vi "FastBeamMode.vi"() -> ()   [LabVIEW 2021]
uses:
  D:/tmytek/Source/bbox-api/example/BBoxOne Series/LabVIEW/BBoxAPI.dll
  BBoxAPI.dll
  Kernel32.dll
panel:
  out "Console Log":string
  out "ScanningDevice":string[](array[string])
  out "Target AAKit Name":string
  out "selectAAKit":i32(ring)=13 items=["OK"=0, "WARNING"=1, "ERROR"=2, "NO_RESPONSE"=3, "ERROR_GET_SN"=10, "ERROR_DEV_TYPE"=11, "ERROR_INIT_OBJECT"=12, "ERROR_DEV_NOT_INIT"=13, "ERROR_METHOD_NOT_FOUND"=14, "ERROR_REFLECTION"=15, "ERROR_POWER"=16, "ERROR_NETWORK_NOT_INIT"=20, "ERROR_NETWORK_INIT"=21, "ERROR_NETWORK_CONNECT_TIMEOUT"=22, "ERROR_DISCONNECT"=23, "ERROR_SOCKET"=24, "ERROR_SEND_CMD"=25, "ERROR_RESP_CMD"=26, "ERROR_DEV_COUNT_ZERO"=30, "ERROR_CMD"=40, "ERROR_CMD_INIT"=41, "ERROR_BF_AAKIT"=100, "ERROR_BF_NO_AAKIT"=101, "ERROR_BF_CALI_PATH"=102, "ERROR_BF_BEAMXY"=103, "ERROR_BF_GEN"=104, "ERROR_BF_TRMODE"=105, "STATUS_BF_LOAD_CALI_INCOMPLTE"=106, "ERROR_BF_LOAD_CALI_PARSE_FAILED"=107, "ERROR_FREQ_EQUATION"=250, "ERROR_PLO_CRC"=251, "WARNING_HARMONIC"=252, "ERROR_HARMONIC_BLOCK"=253]
  out "checkCaliTableLocation":bool
  in  "Fast BeamMode Enable":bool=TRUE
  out "getAAKitList":string[](array[string])
  out "getFrequencyList":string[](array[string])
  in  "Target AAKit Index":i32 min=1 max=2 step=1
  in  "Target Freq Index":i32 min=1 max=2 step=1
  out "setOperatingFreq":i32(ring)=13 items=["OK"=0, "WARNING"=1, "ERROR"=2, "NO_RESPONSE"=3, "ERROR_GET_SN"=10, "ERROR_DEV_TYPE"=11, "ERROR_INIT_OBJECT"=12, "ERROR_DEV_NOT_INIT"=13, "ERROR_METHOD_NOT_FOUND"=14, "ERROR_REFLECTION"=15, "ERROR_POWER"=16, "ERROR_NETWORK_NOT_INIT"=20, "ERROR_NETWORK_INIT"=21, "ERROR_NETWORK_CONNECT_TIMEOUT"=22, "ERROR_DISCONNECT"=23, "ERROR_SOCKET"=24, "ERROR_SEND_CMD"=25, "ERROR_RESP_CMD"=26, "ERROR_DEV_COUNT_ZERO"=30, "ERROR_CMD"=40, "ERROR_CMD_INIT"=41, "ERROR_BF_AAKIT"=100, "ERROR_BF_NO_AAKIT"=101, "ERROR_BF_CALI_PATH"=102, "ERROR_BF_BEAMXY"=103, "ERROR_BF_GEN"=104, "ERROR_BF_TRMODE"=105, "STATUS_BF_LOAD_CALI_INCOMPLTE"=106, "ERROR_BF_LOAD_CALI_PARSE_FAILED"=107, "ERROR_FREQ_EQUATION"=250, "ERROR_PLO_CRC"=251, "WARNING_HARMONIC"=252, "ERROR_HARMONIC_BLOCK"=253]
  out "SN":string
  out "Set_Fast_Parallel_Mode":i32(ring) items=["OK"=0, "WARNING"=1, "ERROR"=2, "NO_RESPONSE"=3, "ERROR_GET_SN"=10, "ERROR_DEV_TYPE"=11, "ERROR_INIT_OBJECT"=12, "ERROR_DEV_NOT_INIT"=13, "ERROR_METHOD_NOT_FOUND"=14, "ERROR_REFLECTION"=15, "ERROR_POWER"=16, "ERROR_SCAN_NOT_FOUND"=17, "ERROR_UNMATCH_RETURN_TYPE"=18, "ERROR_NETWORK_NOT_INIT"=20, "ERROR_NETWORK_INIT"=21, "ERROR_NETWORK_CONNECT_TIMEOUT"=22, "ERROR_DISCONNECT"=23, "ERROR_SOCKET"=24, "ERROR_SEND_CMD"=25, "ERROR_RESP_CMD"=26, "ERROR_DEV_COUNT_ZERO"=30, "ERROR_DEV_DUMMY_FUNC"=31, "ERROR_CMD"=40, "ERROR_CMD_INIT"=41, "ERROR_BF_AAKIT"=100, "ERROR_BF_NO_AAKIT"=101, "ERROR_BF_CALI_PATH"=102, "ERROR_BF_BEAMXY"=103, "ERROR_BF_GEN"=104, "ERROR_BF_TRMODE"=105, "STATUS_BF_LOAD_CALI_INCOMPLTE"=106, "ERROR_BF_LOAD_CALI_PARSE_FAILED"=107, "ERROR_BF_UNLOAD_CALI"=108, "ERROR_BF_CALI_VERSION_UNSUPPORTED"=109, "ERROR_BF_CALI_DATA_NOT_FOUND"=110, "ERROR_FREQ_EQUATION"=250, "ERROR_PLO_CRC"=251, "WARNING_HARMONIC"=252, "ERROR_HARMONIC_BLOCK"=253, "ERROR_FW_UPGRADE_IP_INVALID"=300, "ERROR_FW_VERSION_NOT_SUPPORT"=301]
  out "Init":i32(ring)=13 items=["OK"=0, "WARNING"=1, "ERROR"=2, "NO_RESPONSE"=3, "ERROR_GET_SN"=10, "ERROR_DEV_TYPE"=11, "ERROR_INIT_OBJECT"=12, "ERROR_DEV_NOT_INIT"=13, "ERROR_METHOD_NOT_FOUND"=14, "ERROR_REFLECTION"=15, "ERROR_POWER"=16, "ERROR_NETWORK_NOT_INIT"=20, "ERROR_NETWORK_INIT"=21, "ERROR_NETWORK_CONNECT_TIMEOUT"=22, "ERROR_DISCONNECT"=23, "ERROR_SOCKET"=24, "ERROR_SEND_CMD"=25, "ERROR_RESP_CMD"=26, "ERROR_DEV_COUNT_ZERO"=30, "ERROR_CMD"=40, "ERROR_CMD_INIT"=41, "ERROR_BF_AAKIT"=100, "ERROR_BF_NO_AAKIT"=101, "ERROR_BF_CALI_PATH"=102, "ERROR_BF_BEAMXY"=103, "ERROR_BF_GEN"=104, "ERROR_BF_TRMODE"=105, "STATUS_BF_LOAD_CALI_INCOMPLTE"=106, "ERROR_BF_LOAD_CALI_PARSE_FAILED"=107, "ERROR_FREQ_EQUATION"=250, "ERROR_PLO_CRC"=251, "WARNING_HARMONIC"=252, "ERROR_HARMONIC_BLOCK"=253]
  in  "Start":bool=TRUE
  in  "Set Current Working Directory":path
  out "Get Current Working Directory":path
  out "Exists Table Filenames":string[](array[string])
  # "Notice:\n\nThe Set / Get Current Working Diectory Path must be the sample code directory path : bbox-api\\example\\BBoxOne Series\\LabVIEW\\\n\nMust exist\n\n1. bbox-api\\example\\BBoxOne Series\\LabVIEW\\BBoxAPI.dll\n\n2. bbox-api\\example\\BBoxOne Series\\LabVIEW\\files\\\n\n3. bbox-api\\example\\BBoxOne Series\\LabVIEW\\logs\\"
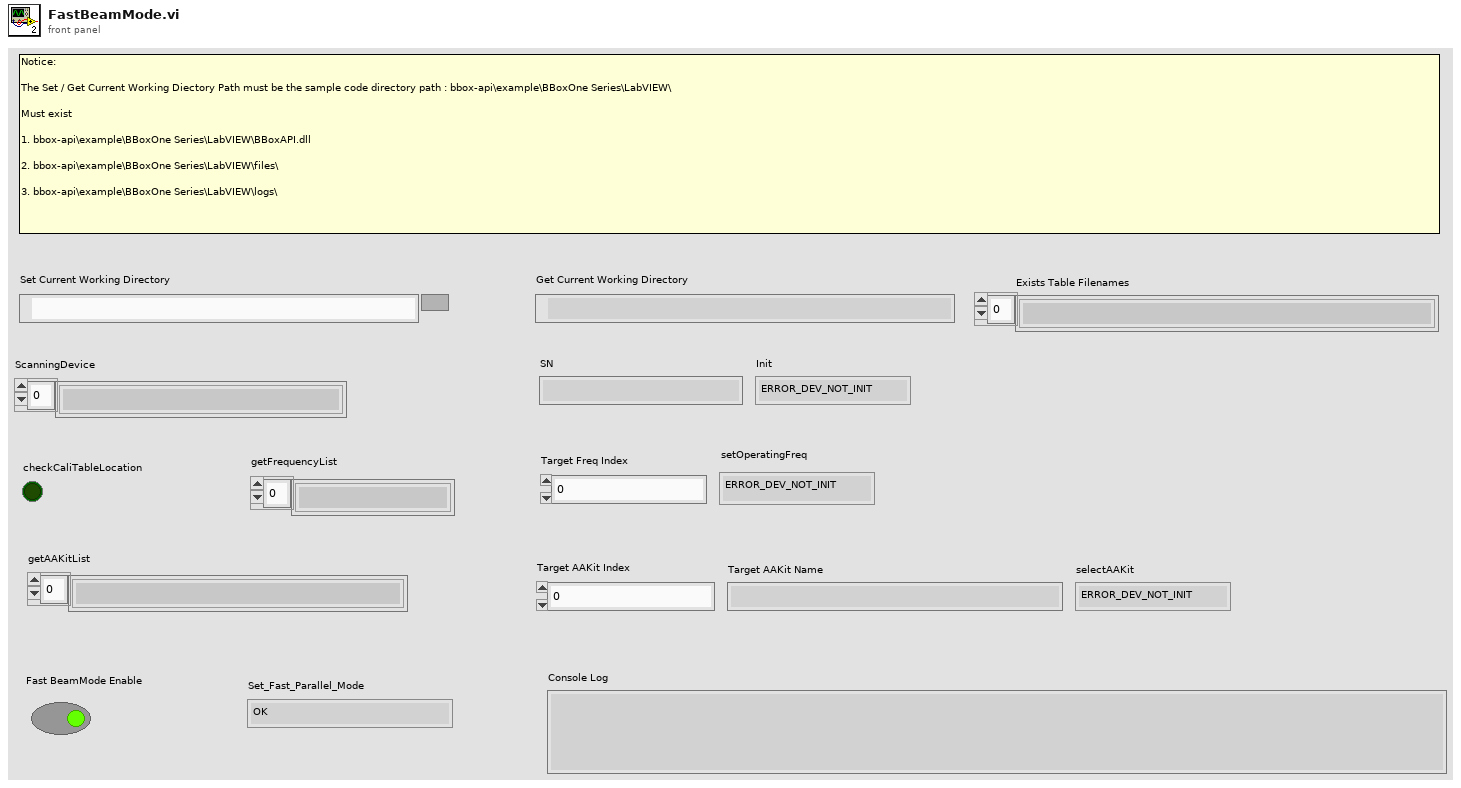
[diagram p1: front panel]
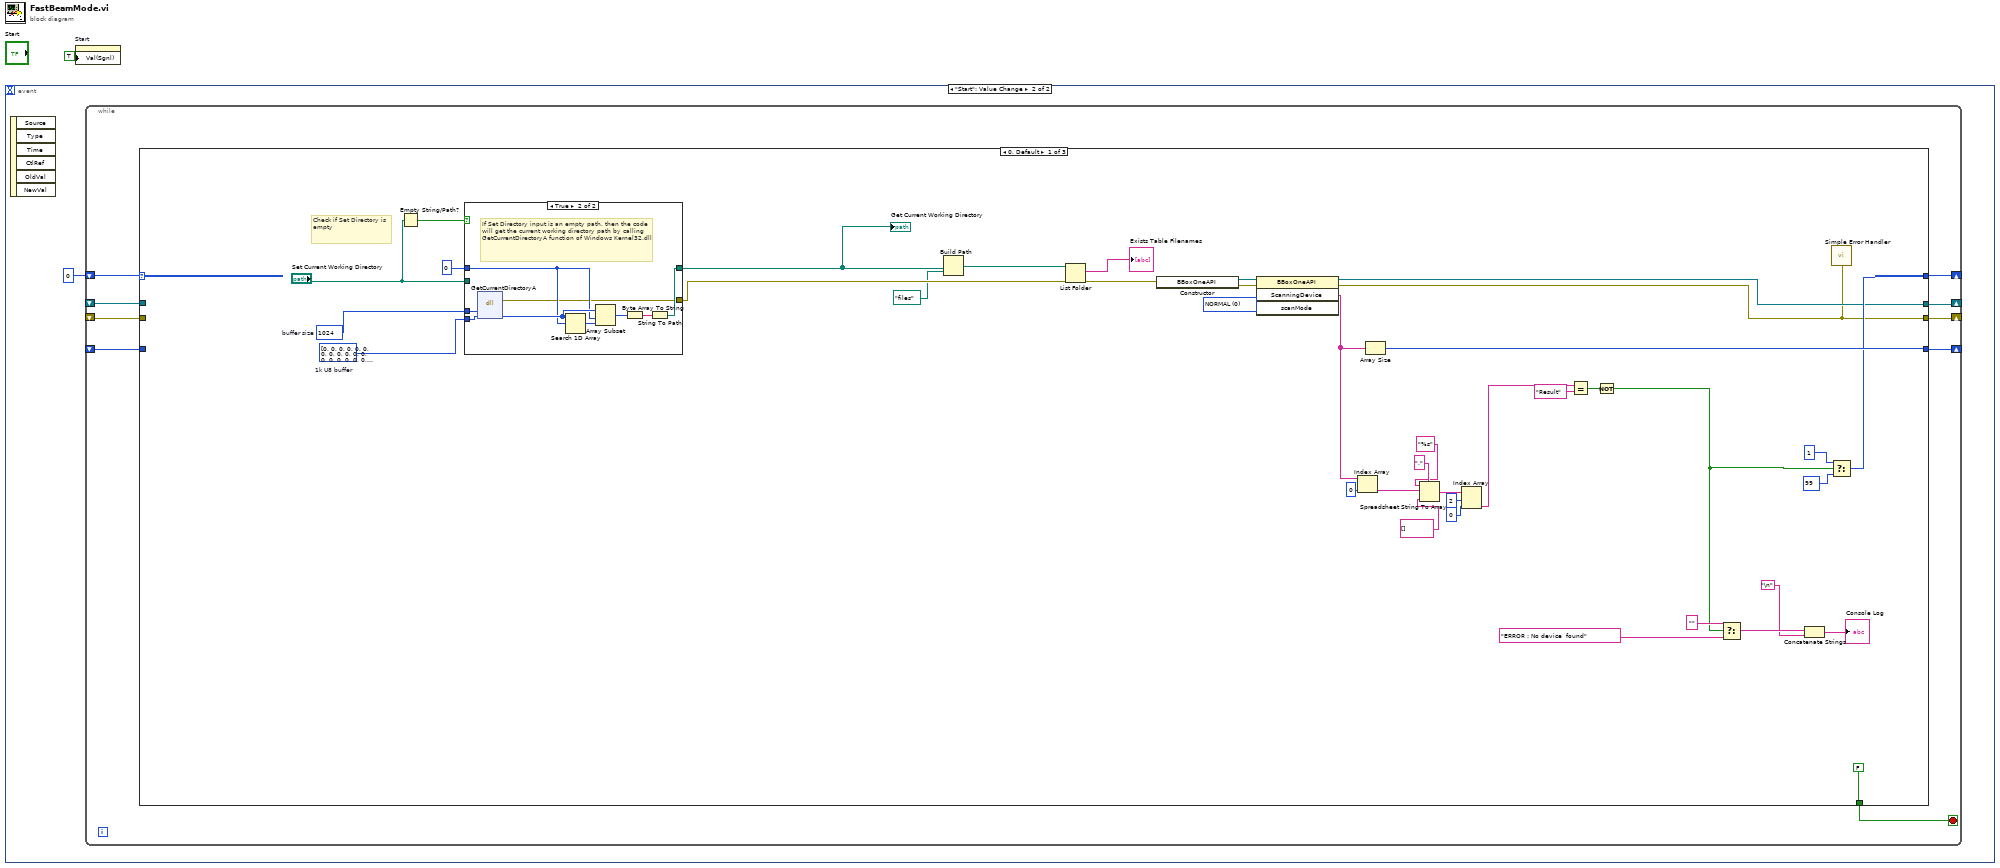
[diagram p0: block diagram]
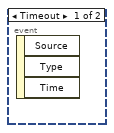
[diagram p2: hidden frame]
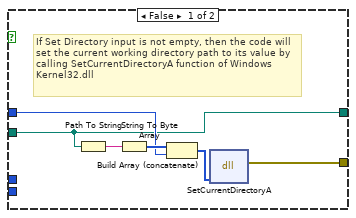
[diagram p3: hidden frame]
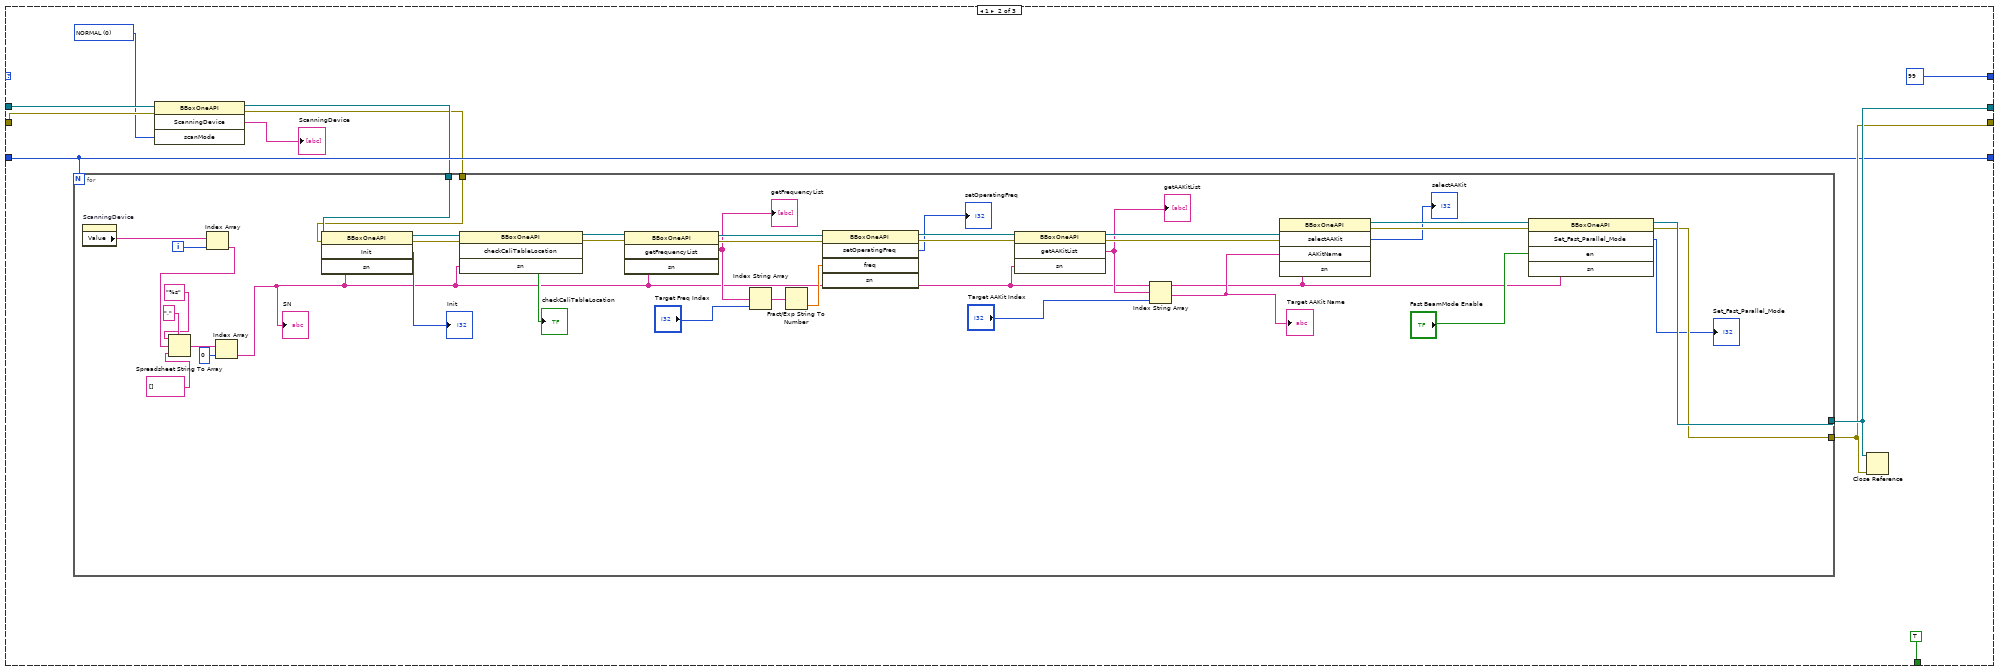
[diagram p4: hidden frame]
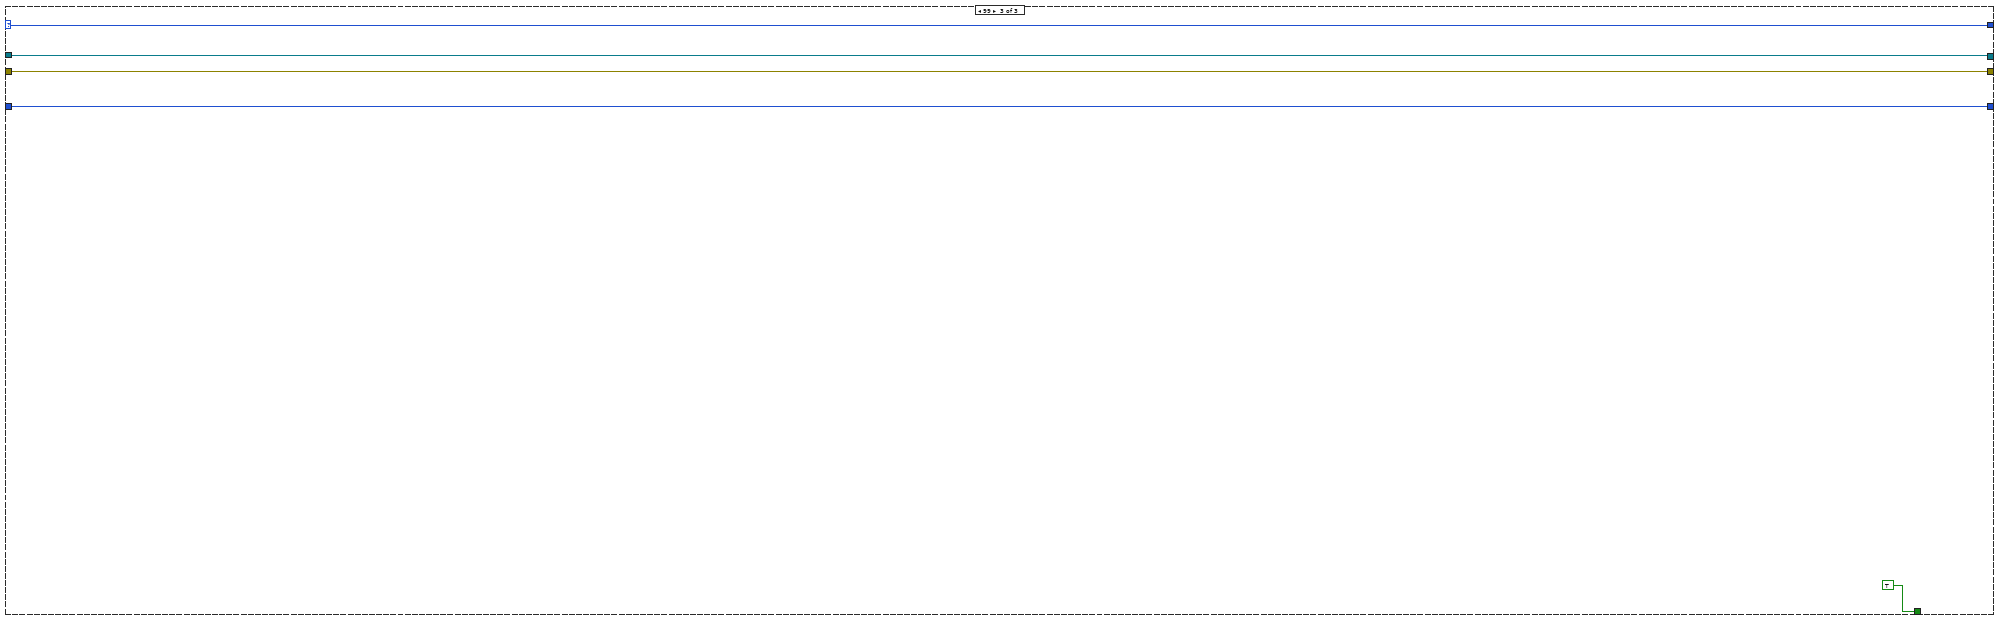
[diagram p5: hidden frame]
diagram:
  n1 = event shown="[1] \"Start\": Value Change" {
    selector: _ -> [_ _]
    dyn-events: _ -> [_ _]
    timeout: _ -> [_ _]
    event Timeout {
      n2 = event-data() -> ()  [unwired: 1 in, 3 out]
    }
    event "Start": Value Change {
      n3 = event-data() -> ()  [unwired: 1 in, 6 out]
      n4 = while {
        shift-right: [w10] -> _
        shift-left: 0 -> [w11]
        shift-right: [w8] -> _
        shift-left: _ -> [w7]
        shift-right: [w6] -> _
        shift-left: _ -> [w3]
        shift-right: [w5] -> _
        shift-left: _ -> [w4]
        stop <- w9 stop-if-true
        n5 = case shown="0, Default" w11 {
          selector: w11 -> [_ _ w119]
          tunnel: [w32 99 w119] -> w10
          tunnel: [FALSE TRUE TRUE] -> w9
          tunnel: [w35 w74 w115] -> w8
          tunnel: w7 -> [_ w74 w115]
          tunnel: [w13 w75 w116] -> w6
          tunnel: [w14 w76 w117] -> w5
          tunnel: w4 -> [_ w71 w117]
          tunnel: w3 -> [_ w70 w116]
          frame 0, Default {
            w42 = 1024  # buffer size
            w41 = u8[] [0, 0, 0, 0, 0, 0, 0, 0, 0, 0, 0, 0, 0, 0, 0, 0, 0, 0, 0, 0, 0, 0, 0, 0, 0, 0, 0, 0, 0, 0, 0, 0, 0, 0, 0, 0, 0, 0, 0, 0, 0, 0, 0, 0, 0, 0, 0, 0, 0, 0, 0, 0, 0, 0, 0, 0, 0, 0, 0, 0, 0, 0, 0, 0, 0, 0, 0, 0, 0, 0, 0, 0, 0, 0, 0, 0, 0, 0, 0, 0, 0, 0, 0, 0, 0, 0, 0, 0, 0, 0, 0, 0, 0, 0, 0, 0, 0, 0, 0, 0, 0, 0, 0, 0, 0, 0, 0, 0, 0, 0, 0, 0, 0, 0, 0, 0, 0, 0, 0, 0, 0, 0, 0, 0, 0, 0, 0, 0, 0, 0, 0, 0, 0, 0, 0, 0, 0, 0, 0, 0, 0, 0, 0, 0, 0, 0, 0, 0, 0, 0, 0, 0, 0, 0, 0, 0, 0, 0, 0, 0, 0, 0, 0, 0, 0, 0, 0, 0, 0, 0, 0, 0, 0, 0, 0, 0, 0, 0, 0, 0, 0, 0, 0, 0, 0, 0, 0, 0, 0, 0, 0, 0, 0, 0, 0, 0, 0, 0, 0, 0, 0, 0, 0, 0, 0, 0, 0, 0, 0, 0, 0, 0, 0, 0, 0, 0, 0, 0, 0, 0, 0, 0, 0, 0, 0, 0, 0, 0, 0, 0, 0, 0, 0, 0, 0, 0, 0, 0, 0, 0, 0, 0, 0, 0, 0, 0, 0, 0, 0, 0, 0, 0, 0, 0, 0, 0, 0, 0, 0, 0, 0, 0, 0, 0, 0, 0, 0, 0, 0, 0, 0, 0, 0, 0, 0, 0, 0, 0, 0, 0, 0, 0, 0, 0, 0, 0, 0, 0, 0, 0, 0, 0, 0, 0, 0, 0, 0, 0, 0, 0, 0, 0, 0, 0, 0, 0, 0, 0, 0, 0, 0, 0, 0, 0, 0, 0, 0, 0, 0, 0, 0, 0, 0, 0, 0, 0, 0, 0, 0, 0, 0, 0, 0, 0, 0, 0, 0, 0, 0, 0, 0, 0, 0, 0, 0, 0, 0, 0, 0, 0, 0, 0, 0, 0, 0, 0, 0, 0, 0, 0, 0, 0, 0, 0, 0, 0, 0, 0, 0, 0, 0, 0, 0, 0, 0, 0, 0, 0, 0, 0, 0, 0, 0, 0, 0, 0, 0, 0, 0, 0, 0, 0, 0, 0, 0, 0, 0, 0, 0, 0, 0, 0, 0, 0, 0, 0, 0, 0, 0, 0, 0, 0, 0, 0, 0, 0, 0, 0, 0, 0, 0, 0, 0, 0, 0, 0, 0, 0, 0, 0, 0, 0, 0, 0, 0, 0, 0, 0, 0, 0, 0, 0, 0, 0, 0, 0, 0, 0, 0, 0, 0, 0, 0, 0, 0, 0, 0, 0, 0, 0, 0, 0, 0, 0, 0, 0, 0, 0, 0, 0, 0, 0, 0, 0, 0, 0, 0, 0, 0, 0, 0, 0, 0, 0, 0, 0, 0, 0, 0, 0, 0, 0, 0, 0, 0, 0, 0, 0, 0, 0, 0, 0, 0, 0, 0, 0, 0, 0, 0, 0, 0, 0, 0, 0, 0, 0, 0, 0, 0, 0, 0, 0, 0, 0, 0, 0, 0, 0, 0, 0, 0, 0, 0, 0, 0, 0, 0, 0, 0, 0, 0, 0, 0, 0, 0, 0, 0, 0, 0, 0, 0, 0, 0, 0, 0, 0, 0, 0, 0, 0, 0, 0, 0, 0, 0, 0, 0, 0, 0, 0, 0, 0, 0, 0, 0, 0, 0, 0, 0, 0, 0, 0, 0, 0, 0, 0, 0, 0, 0, 0, 0, 0, 0, 0, 0, 0, 0, 0, 0, 0, 0, 0, 0, 0, 0, 0, 0, 0, 0, 0, 0, 0, 0, 0, 0, 0, 0, 0, 0, 0, 0, 0, 0, 0, 0, 0, 0, 0, 0, 0, 0, 0, 0, 0, 0, 0, 0, 0, 0, 0, 0, 0, 0, 0, 0, 0, 0, 0, 0, 0, 0, 0, 0, 0, 0, 0, 0, 0, 0, 0, 0, 0, 0, 0, 0, 0, 0, 0, 0, 0, 0, 0, 0, 0, 0, 0, 0, 0, 0, 0, 0, 0, 0, 0, 0, 0, 0, 0, 0, 0, 0, 0, 0, 0, 0, 0, 0, 0, 0, 0, 0, 0, 0, 0, 0, 0, 0, 0, 0, 0, 0, 0, 0, 0, 0, 0, 0, 0, 0, 0, 0, 0, 0, 0, 0, 0, 0, 0, 0, 0, 0, 0, 0, 0, 0, 0, 0, 0, 0, 0, 0, 0, 0, 0, 0, 0, 0, 0, 0, 0, 0, 0, 0, 0, 0, 0, 0, 0, 0, 0, 0, 0, 0, 0, 0, 0, 0, 0, 0, 0, 0, 0, 0, 0, 0, 0, 0, 0, 0, 0, 0, 0, 0, 0, 0, 0, 0, 0, 0, 0, 0, 0, 0, 0, 0, 0, 0, 0, 0, 0, 0, 0, 0, 0, 0, 0, 0, 0, 0, 0, 0, 0, 0, 0, 0, 0, 0, 0, 0, 0, 0, 0, 0, 0, 0, 0, 0, 0, 0, 0, 0, 0, 0, 0, 0, 0, 0, 0, 0, 0, 0, 0, 0, 0, 0, 0, 0, 0, 0, 0, 0, 0, 0, 0, 0, 0, 0, 0, 0, 0, 0, 0, 0, 0, 0, 0, 0, 0, 0, 0, 0, 0, 0, 0, 0, 0, 0, 0, 0, 0, 0, 0, 0, 0, 0, 0, 0, 0, 0, 0, 0, 0, 0, 0, 0, 0, 0, 0, 0, 0, 0, 0, 0, 0, 0, 0, 0, 0, 0, 0, 0, 0, 0, 0, 0, 0, 0, 0, 0, 0, 0, 0, 0, 0, 0, 0, 0, 0, 0, 0, 0, 0, 0, 0, 0, 0, 0, 0, 0, 0, 0, 0, 0, 0, 0, 0, 0, 0, 0, 0, 0, 0, 0, 0, 0, 0, 0, 0, 0, 0, 0, 0, 0, 0, 0, 0, 0, 0, 0, 0, 0, 0, 0, 0, 0, 0, 0, 0, 0, 0, 0, 0, 0, 0, 0, 0, 0, 0, 0, 0, 0, 0, 0, 0, 0, 0, 0, 0, 0, 0, 0, 0, 0, 0, 0, 0, 0, 0, 0, 0, 0, 0, 0, 0, 0, 0, 0, 0, 0, 0, 0, 0, 0, 0]  # 1k U8 buffer
            w40 = 0 items=["NORMAL", "FAST"] ("scanMode")
            # "Check if Set Directory is empty"
            n6 = Empty String/Path?(string/path="Set Current Working Directory") -> (empty?=w47:bool)
            n7 = case shown="True" w47 {
              tunnel: "Set Current Working Directory" -> [w52 _]
              tunnel: u8 0 -> [w54 w61]
              tunnel: w42 -> [_ w60]
              tunnel: w41 -> [_ w59]
              tunnel: [w52 w58] -> w36
              tunnel: [w51 w57] -> w49
              frame False {
                # "If Set Directory input is not empty, then the code will set the current working directory path to its value by calling SetCurrentDirectoryA function of Windows Kernel32.dll"
                n8 = Path To String(path=w52) -> (string=w53:string)
                n9 = String To Byte Array(string=w53) -> (unsigned byte array=w56:u8[])
                n10 = Build Array (concatenate)(w56, w54) -> (w55:u8[])
                n11 = dll-call lib="Kernel32.dll" fn="SetCurrentDirectoryA" label="Kernel32.dll - \nSetCurrentDirectoryA"("lpPathName"=w55) -> (error out=w51:errorcluster)  [unwired: 4 in, 2 out]
              }
              frame True {
                # "If Set Directory input is an empty path, then the code will get the current working directory path by calling GetCurrentDirectoryA function of Windows Kernel32.dll"
                n12 = dll-call lib="kernel32.dll" fn="GetCurrentDirectoryA" label="Kernel32.dll - \nGetCurrentDirectoryA"("nBufferLength"=w60, "lpBuffer"=w59) -> (error out=w57:errorcluster, "lpBuffer"=w64:u8[])  [unwired: 4 in, 2 out]
                n13 = Search 1D Array(1D array=w64, element=w61) -> (index of element=w65:i32)  [unwired: 1 out]
                n14 = Array Subset(array=w64, index=w61, length=w65) -> (w62:u8[])
                n15 = Byte Array To String(unsigned byte array=w62) -> (string=w63:string)
                n16 = String To Path(string=w63) -> (path=w58:path)
              }
            }
            "Get Current Working Directory" <- w36
            n17 = Build Path(base path=w36, name or relative path=path "files") -> (appended path=w48:path)
            n18 = List Folder(path=w48, error in=w49) -> (filenames=→"Exists Table Filenames":string[], error out=w50:errorcluster)  [unwired: 2 in, 2 out]
            n19 = constructor class="BBoxOneAPI"(error in=w50) -> (reference out=w45:refnum<k24>, error out=w46:errorcluster)  [unwired: 2 in, 1 out]
            n20 = invoke class="BBoxOneAPI" method="ScanningDevice"(reference=w45, error in=w46, "scanMode"=w40) -> (reference out=w14:refnum<k24>, error out=w13:errorcluster, "ScanningDevice"=w15:string[])  [unwired: 1 in, 1 out]
            n21 = Index Array(array=w15, index=0) -> (element=w28:string)
            n22 = Array Size(array=w15) -> (size(s)=w35:i32)
            n23 = Spreadsheet String To Array(delimiter (Tab)=",", format string="%s", spreadsheet string=w28, array type (2D Dbl)=string[] []) -> (array=w26:string[])
            n24 = Index Array(array=w26, index #1=2 ("index"), index #2=0 ("index")) -> (element #2=w17:string)  [unwired: 1 out]
            n25 = Equal?(x=w17, y="Result") -> (x = y?=w18:bool)
            n26 = Not(x=w18) -> (.not. x?=w12:bool)
            n27 = Select(t="" ("y"), s=w12, f="ERROR : No device  found" ("y")) -> (s? t:f=w20:string)
            n28 = Concatenate Strings(w20, "\n") -> (→"Console Log":string)
            n29 = call <vilib>:"Simple Error Handler.vi"("error in (no error)"=w13) -> ()  [unwired: 4 in, 5 out]
            n30 = Select(t=1, s=w12, f=99) -> (s? t:f=w32:i32)
          }
          frame 1 {
            w67 = 0 items=["NORMAL", "FAST", "ETH_DISABLE"] ("scanMode")
            n31 = invoke class="BBoxOneAPI" method="ScanningDevice"(reference=w71, error in=w70, "scanMode"=w67) -> (reference out=w69:refnum<k24>, error out=w68:errorcluster, "ScanningDevice"=→"ScanningDevice":string[])  [unwired: 1 in, 1 out]
            n32 = for {
              N: w74 -> [_]
              tunnel: w69 -> [w114]
              tunnel: w68 -> [w113]
              tunnel: [w100] -> w75
              tunnel: [w101] -> w76
              i -> [w106]
              n33 = property on="ScanningDevice" class="Arr (strict)"() -> ("Value"=w84:string[])  [unwired: 2 in, 2 out]
              n34 = Index Array(array=w84, index=w106) -> (element=w78:string)
              n35 = Spreadsheet String To Array(delimiter (Tab)=",", format string="%s", spreadsheet string=w78, array type (2D Dbl)=string[] []) -> (array=w80:string[])
              n36 = Index Array(array=w80, index=0) -> (element=w77:string)
              "SN" <- w77
              n37 = invoke class="BBoxOneAPI" method="Init"(reference=w114, error in=w113, "sn"=w77) -> (reference out=w99:refnum<k24>, error out=w98:errorcluster, "Init"=→"Init":i32)  [unwired: 1 in, 1 out]
              n38 = invoke class="BBoxOneAPI" method="checkCaliTableLocation"(reference=w99, error in=w98, "sn"=w77) -> (reference out=w97:refnum<k24>, error out=w96:errorcluster, "checkCaliTableLocation"=→"checkCaliTableLocation":bool)  [unwired: 1 in, 1 out]
              n39 = invoke class="BBoxOneAPI" method="getFrequencyList"(reference=w97, error in=w96, "sn"=w77) -> (reference out=w108:refnum<k24>, error out=w107:errorcluster, "getFrequencyList"=w91:string[])  [unwired: 1 in, 1 out]
              "getFrequencyList" <- w91
              n40 = Index String Array(1:"Target Freq Index", 2:w91) -> (0:w105:string)  [unwired: 1 in]
              n41 = Fract/Exp String To Number(string=w105) -> (number=w104:dbl)  [unwired: 3 in, 1 out]
              n42 = invoke class="BBoxOneAPI" method="setOperatingFreq"(reference=w108, error in=w107, "freq"=w104, "sn"=w77) -> (reference out=w112:refnum<k24>, error out=w111:errorcluster, "setOperatingFreq"=→"setOperatingFreq":i32)  [unwired: 1 in, 2 out]
              n43 = invoke class="BBoxOneAPI" method="getAAKitList"(reference=w112, error in=w111, "sn"=w77) -> (reference out=w110:refnum<k24>, error out=w109:errorcluster, "getAAKitList"=w90:string[])  [unwired: 1 in, 1 out]
              "getAAKitList" <- w90
              n44 = Index String Array(1:"Target AAKit Index", 2:w90) -> (0:w86:string)  [unwired: 1 in]
              "Target AAKit Name" <- w86
              n45 = invoke class="BBoxOneAPI" method="selectAAKit"(reference=w110, error in=w109, "AAKitName"=w86, "sn"=w77) -> (reference out=w103:refnum<k24>, error out=w102:errorcluster, "selectAAKit"=→"selectAAKit":i32)  [unwired: 1 in, 2 out]
              n46 = invoke class="BBoxOneAPI" method="Set_Fast_Parallel_Mode"(reference=w103, error in=w102, "en"="Fast BeamMode Enable", "sn"=w77) -> (reference out=w101:refnum<k24>, error out=w100:errorcluster, "Set_Fast_Parallel_Mode"=→"Set_Fast_Parallel_Mode":i32)  [unwired: 1 in, 2 out]
            }
            n47 = Close Reference(reference=w76, error in (no error)=w75) -> ()  [unwired: 1 out]
          }
          frame 99 {
          }
        }
      }
    }
  }
  n48 = property on="Start" class="Bool (strict)"("Val(Sgnl)"=TRUE ("Value (Signaling)")) -> ()  [unwired: 2 in, 2 out]
